vi "ForLoop.vi"() -> ()   [LabVIEW 2020]
panel:
  out "milliseconds to wait 2":u32
  in  "milliseconds to wait":u32
  out "Numeric 2":i32
  in  "stop":bool
  in  "Numeric":i32
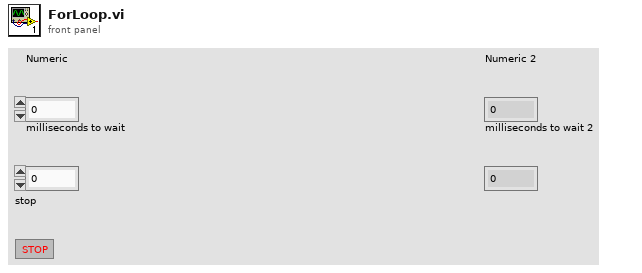
[diagram p1: front panel]
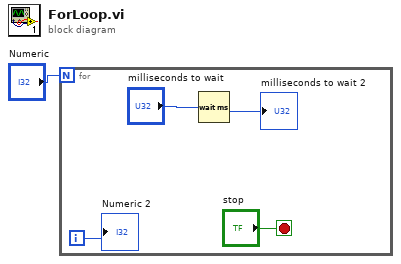
[diagram p0: block diagram]
diagram:
  n1 = for {
    N: "Numeric" -> [_]
    i -> [w4]
    stop <- "stop" stop-if-true
    n2 = Wait (ms)(milliseconds to wait="milliseconds to wait") -> (millisecond timer value=→"milliseconds to wait 2":u32)
    "Numeric 2" <- w4
  }
